vi "DrawScore.vi"(5 "Digits":i32, 6 "AutoWidth?":bool, 7 "Color":T2, 8 "error in (no error)":errorcluster, 9 "score":i16, 10 "position":T1, 11 "Pong in":refnum<class "Game.lvclass">) -> (0 "error out":errorcluster, 3 "Pong out":refnum<class "Game.lvclass">)   [LabVIEW 2019, in "RT_Game.lvlib" / "Game.lvclass"]
uses:
  Game.lvclass
  Color.ctl
  Coordinate.ctl
  RT_Game.lvlib
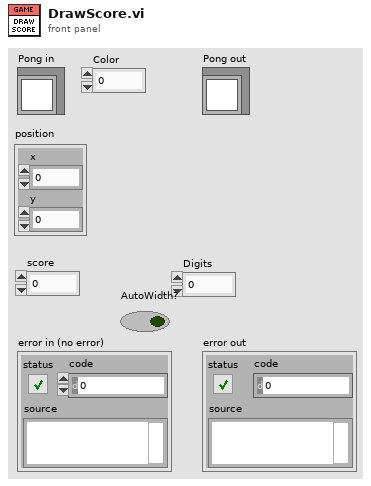
[diagram p1: front panel]
types:
  T1 = typedef "RT_Game.lvlib/Game.lvclass/Coordinate.ctl" = cluster{"x":dbl, "y":dbl}
  T2 = typedef "RT_Game.lvlib/Color.ctl" = fxp<+,3,3>
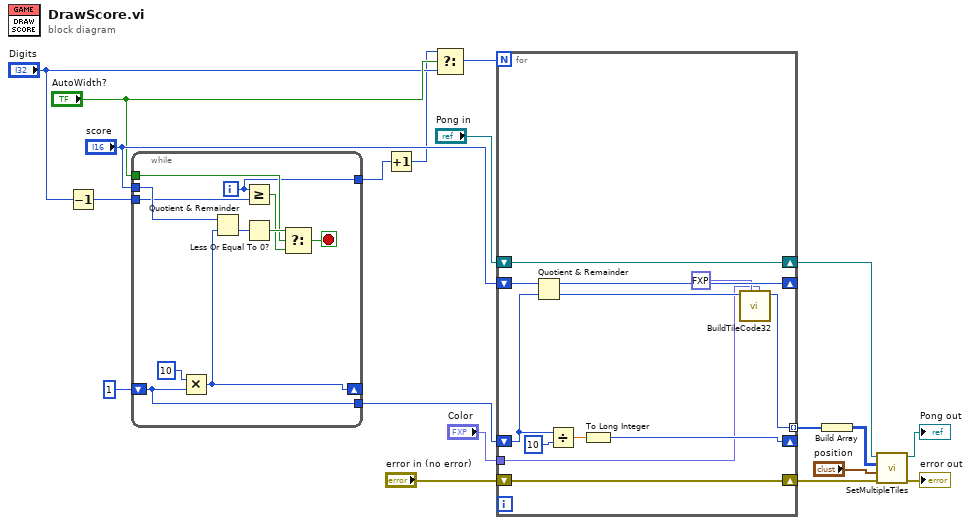
[diagram p0: block diagram]
diagram:
  n1 = Decrement(x="Digits") -> (x-1=w3:i32)
  n2 = while {
    shift-right: [w27] -> _
    shift-left: 1 -> [w28]
    tunnel: [w28] -> w9
    tunnel: "score" -> [w29]
    tunnel: "AutoWidth?" -> [w22]
    tunnel: w3 -> [w23]
    tunnel: [w20] -> w2
    i -> [w20]
    stop <- w24 stop-if-true
    n3 = Multiply(x=10, y=w28) -> (x*y=w27:i32)
    n4 = Quotient & Remainder(x=w29, y=w27) -> (floor(x/y)=w26:i32)  [unwired: 1 out]
    n5 = Greater Or Equal?(x=w20, y=w23) -> (x >= y?=w21:bool)
    n6 = Less Or Equal To 0?(x=w26) -> (x <= 0?=w25:bool)
    n7 = Select(t=w25, s=w22, f=w21) -> (s? t:f=w24:bool)
  }
  n8 = Increment(x=w2) -> (x+1=w1:i32)
  n9 = Select(t=w1, s="AutoWidth?", f="Digits") -> (s? t:f=w6:i32)
  n10 = for {
    N: w6 -> [_]
    shift-right: [w42] -> w16
    shift-left: "error in (no error)" -> [w42]
    shift-right: [w41] -> w17
    shift-left: "Pong in" -> [w41]
    shift-right: [w37] -> _
    shift-left: w9 -> [w40]
    shift-right: [w34] -> _
    shift-left: "score" -> [w35]
    tunnel: "Color" -> [w31]
    tunnel: [w36] -> w18 mode=indexing
    n11 = Quotient & Remainder(x=w35, y=w40) -> (x-y*floor(x/y)=w34:i32, floor(x/y)=w33:i32)
    n12 = Divide(x=w40, y=10) -> (x/y=w38:dbl)
    n13 = To Long Integer(number=w38) -> (32bit integer=w37:i32)
    n14 = call "BuildTileCode32.vi"("replacecolor"=w31, "color_to_replace"=fxp<+,3,3> 7.0, "Tilenumber"=w33) -> ("TileCode"=w36:u32)  [unwired: 8 in]
  }
  n15 = Build Array(w18) -> (w19:u32[][])
  n16 = call "SetMultipleTiles.vi"("error in (no error)"=w16, "Position"="position", "TileCodes"=w19, "Game in"=w17) -> ("error out"=→"error out":errorcluster, "Game out"=→"Pong out":refnum<class "Game.lvclass">)  [unwired: 6 in]
